vi "f_MGCC_PVFcst_ActualPV.vi"() -> ()   [LabVIEW 2016, in "MGCC_PVFcst_dataIO.lvlib"]
uses:
  Lib/MGCC_PVFcst_dataIO.lvlib
panel:
  in  "ActualPV":dbl[](array[numeric])
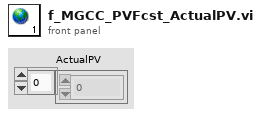
[diagram p1: front panel]
diagram:
